vi "HW_Gantner_Concatenant Data.vi"() -> ()   [LabVIEW 2016]
panel:
  out "data out":waveform(dbl)[](array[waveform])
  in  "data in":waveform(dbl)[](array[waveform])
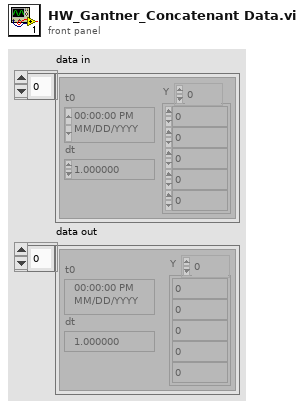
[diagram p1: front panel]
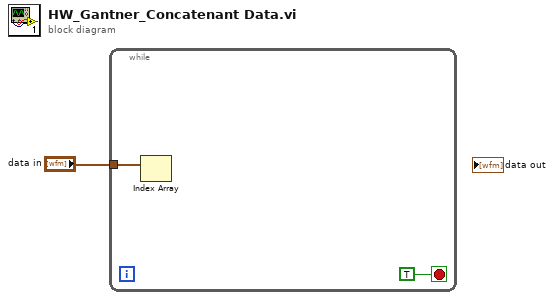
[diagram p0: block diagram]
diagram:
  n1 = while {
    tunnel: "data in" -> [w2]
    stop <- TRUE stop-if-true
    n2 = Index Array(array=w2) -> ()  [unwired: 1 in, 1 out]
  }
